vi "st_Binomial Inverse CDF (kx).vi"(9 "p":dbl=0.1, 10 "n":i32=100, 11 "cdf(x)":dbl=0.5) -> (0 "error":i32, 3 "x":dbl=0.5)   [LabVIEW 2020, in "NI_Gmath.lvlib"]
uses:
  <vilib>/gmath/NI_Gmath.lvlib
  <vilib>/gmath/statdist.llb/st_error_code.ctl
panel:
  # "Binomial Inverse CDF"
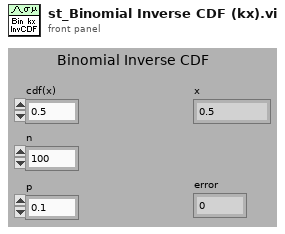
[diagram p1: front panel]
types:
  T1 = typedef "NI_Gmath.lvlib/st_error_code.ctl" = i32
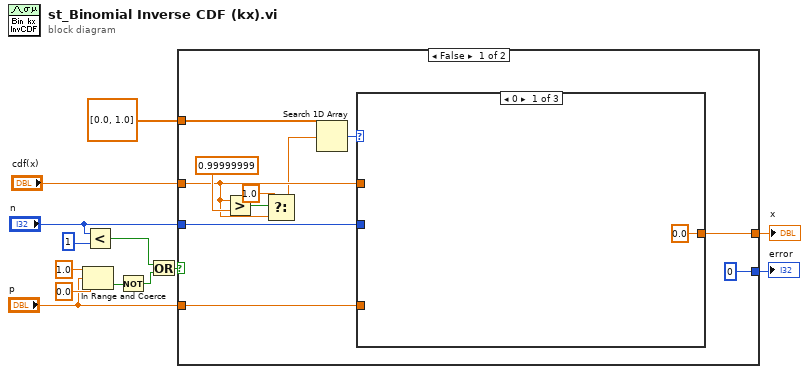
[diagram p0: block diagram]
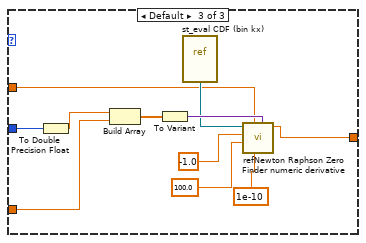
[diagram p3: hidden frame]
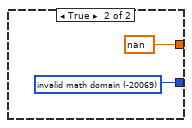
[diagram p4: hidden frame]
diagram:
  n1 = In Range and Coerce(upper limit=1.0, x="p", lower limit=0.0) -> (In Range?=w8:bool)  [unwired: 1 out]
  n2 = Less?(x="n", y=1) -> (x < y?=w6:bool)
  n3 = Not(x=w8) -> (.not. x?=w7:bool)
  n4 = Or(x=w6, y=w7) -> (x .or. y?=w2:bool)
  n5 = case shown="False" w2 {
    tunnel: "p" -> [w21 _]
    tunnel: [0 ("invalid math domain") w38] -> w13
    tunnel: [w22 nan] -> w12
    tunnel: "cdf(x)" -> [w16 _]
    tunnel: "n" -> [w23 _]
    tunnel: dbl[] [0.0, 1.0] -> [w20 _]
    frame False {
      n6 = Greater?(x=w16, y=0.99999999) -> (0:w17:bool)
      n7 = Select(t=1.0, s=w17, f=w16) -> (s? t:f=w14:dbl)
      n8 = Search 1D Array(1D array=w20, element=w14) -> (index of element=w19:i32)  [unwired: 1 in]
      n9 = case shown="0" w19 {
        tunnel: w23 -> [_ w26 w35]
        tunnel: w21 -> [_ _ w34]
        tunnel: [0.0 ("zero") w26 w33] -> w22
        tunnel: w16 -> [_ _ w31]
        frame 0 {
        }
        frame 1 {
        }
        frame Default {
          n10 = To Double Precision Float(number=w35) -> (double precision float=w27:dbl)
          n11 = Build Array(w27, w34) -> (w37:dbl[])
          n12 = To Variant(anything=w37) -> (Variant=w36:variant)
          n13 = vi-ref <vilib>:"st_eval CDF (bin kx).vi"() -> ("vi reference"=w32:refnum<vi>)
          n14 = call <vilib>:"refNewton Raphson Zero Finder numeric derivative.vi"("function parameters"=w36, "accuracy"=1e-10, "level"=w31, "end"=100.0, "start"=-1.0, "function refnum"=w32) -> ("zero"=w33:dbl)  [unwired: 2 in, 3 out]
        }
      }
    }
    frame True {
      w38 = T1 -20069 items=["invalid math domain"=-20069, "Fourier interpolation size m >= n"=-20070, "empty array"=-20003] ("stat interp error code")
    }
  }
  "x" <- w12
  "error" <- w13
